vi "Send Command.vi"(8 "Parameters":u8[](array[numeric]), 9 "Command Type":u8, 10 "Command Class":T1, 11 "Port":i32) -> (3 "Port":i32)   [LabVIEW 2010]
uses:
  Command Classes.ctl
  LvSerial/LvSerial.llb/LvSerial.lvlib
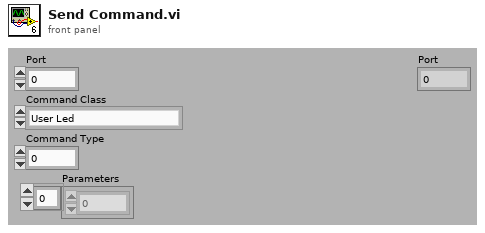
[diagram p1: front panel]
types:
  T1 = typedef "Command Classes.ctl" = enum8{"User Led", "Protocol"}
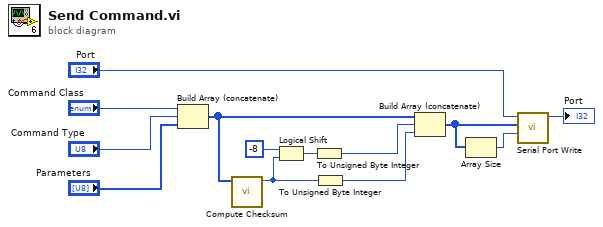
[diagram p0: block diagram]
diagram:
  n1 = Build Array (concatenate)("Command Class", "Command Type", "Parameters") -> (w10:u8[])
  n2 = call "Compute Checksum.vi"("Command"=w10) -> ("Checksum"=w4:u16)  [unwired: 10 in]
  n3 = Logical Shift(y=-8, x=w4) -> (x << y=w1:u16)
  n4 = To Unsigned Byte Integer(number=w1) -> (unsigned 8bit integer=w2:u8)
  n5 = To Unsigned Byte Integer(number=w4) -> (unsigned 8bit integer=w3:u8)
  n6 = Build Array (concatenate)(w10, w2, w3) -> (w7:u8[])
  n7 = Array Size(array=w7) -> (size(s)=w6:i32)
  n8 = call "Serial Port Write.vi"("Length"=w6, "Buffer"=w7, "Port"="Port") -> ("Port"=→"Port":i32)  [unwired: 8 in]
